vi "Serialize ADAS Data.vi"   [LabVIEW 2020]
uses:
  <vilib>/ADAS Record/CustomDataTypes/ADAS Generic/NI_ADAS_Generic.lvlib
  <vilib>/ADAS Record/CustomDataTypes/Ethernet Type 1/NI_ADAS_Ethernet.lvlib
  <vilib>/ADAS Record/CustomDataTypes/Vision Type 1/NI_ADAS_IMAQ_Array.lvlib
  <vilib>/ADAS Record/CustomDataTypes/CAN/NI_ADAS_CAN.lvlib
  <vilib>/ADAS Record/CustomDataTypes/Audio Data/Audio Data.lvlib
  <vilib>/ADAS Record/CustomDataTypes/Byte Array/Byte Array.lvlib
  <vilib>/ADAS Record/CustomDataTypes/Byte Array EDVR/Byte Array EDVR.lvlib
  <vilib>/ADAS Record/CustomDataTypes/Double/Double.lvlib
  <vilib>/ADAS Record/CustomDataTypes/Ethernet Frame/Ethernet Frame.lvlib
  <vilib>/ADAS Record/CustomDataTypes/Extended (EXT)/Extended (EXT).lvlib
  <vilib>/ADAS Record/CustomDataTypes/LIN Frame Array/LIN Frame Array.lvlib
  <vilib>/ADAS Record/CustomDataTypes/Signed Byte (I8)/Signed Byte (I8).lvlib
  <vilib>/ADAS Record/CustomDataTypes/Signed Long (I32)/Signed Long (I32).lvlib
  <vilib>/ADAS Record/CustomDataTypes/Signed Quad (I64)/Signed Quad (I64).lvlib
  <vilib>/ADAS Record/CustomDataTypes/Signed Word (I16)/Signed Word (I16).lvlib
  <vilib>/ADAS Record/CustomDataTypes/Single/Single.lvlib
  <vilib>/ADAS Record/CustomDataTypes/String/String.lvlib
  <vilib>/ADAS Record/CustomDataTypes/Unsigned Byte (U8)/Unsigned Byte (U8).lvlib
  <vilib>/ADAS Record/CustomDataTypes/Unsigned Long (U32)/Unsigned Long (U32).lvlib
  <vilib>/ADAS Record/CustomDataTypes/Unsigned Quad (U64)/Unsigned Quad (U64).lvlib
  <vilib>/ADAS Record/CustomDataTypes/Unsigned Word (U16)/Unsigned Word (U16).lvlib
  <vilib>/ADAS Record/CustomDataTypes/Integer Waveform (U8)/Integer Waveform (U8).lvlib
  <vilib>/ADAS Record/CustomDataTypes/GPS/GPS.lvlib
  <vilib>/ADAS Record/CustomDataTypes/Waveform(DBL) Array/Waveform(DBL) Array.lvlib
  <vilib>/ADAS Record/CustomDataTypes/Boolean/Boolean.lvlib
  <vilib>/ADAS Record/CustomDataTypes/CameraLLPPacketFIFO/CameraLLPPacketFIFO.lvlib
  <vilib>/ADAS Record/CustomDataTypes/Optitrack/Optitrack.lvlib
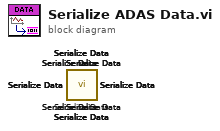
[diagram p0: block diagram]
diagram:
  n1 = call <vilib>:"Serialize Data.vi"() -> ()  [unwired: 10 in, 2 out]
  n2 = call <vilib>:"Serialize Data.vi"() -> ()  [unwired: 10 in, 2 out]
  n3 = call <vilib>:"Serialize Data.vi"() -> ()  [unwired: 10 in, 2 out]
  n4 = call <vilib>:"Serialize Data.vi"() -> ()  [unwired: 10 in, 2 out]
  n5 = call <vilib>:"Serialize Data.vi"() -> ()  [unwired: 10 in, 2 out]
  n6 = call <vilib>:"Serialize Data.vi"() -> ()  [unwired: 10 in, 2 out]
  n7 = call <vilib>:"Serialize Data.vi"() -> ()  [unwired: 10 in, 2 out]
  n8 = call <vilib>:"Serialize Data.vi"() -> ()  [unwired: 10 in, 2 out]
  n9 = call <vilib>:"Serialize Data.vi"() -> ()  [unwired: 10 in, 2 out]
  n10 = call <vilib>:"Serialize Data.vi"() -> ()  [unwired: 10 in, 2 out]
  n11 = call <vilib>:"Serialize Data.vi"() -> ()  [unwired: 10 in, 2 out]
  n12 = call <vilib>:"Serialize Data.vi"() -> ()  [unwired: 10 in, 2 out]
  n13 = call <vilib>:"Serialize Data.vi"() -> ()  [unwired: 10 in, 2 out]
  n14 = call <vilib>:"Serialize Data.vi"() -> ()  [unwired: 10 in, 2 out]
  n15 = call <vilib>:"Serialize Data.vi"() -> ()  [unwired: 10 in, 2 out]
  n16 = call <vilib>:"Serialize Data.vi"() -> ()  [unwired: 10 in, 2 out]
  n17 = call <vilib>:"Serialize Data.vi"() -> ()  [unwired: 10 in, 2 out]
  n18 = call <vilib>:"Serialize Data.vi"() -> ()  [unwired: 10 in, 2 out]
  n19 = call <vilib>:"Serialize Data.vi"() -> ()  [unwired: 10 in, 2 out]
  n20 = call <vilib>:"Serialize Data.vi"() -> ()  [unwired: 10 in, 2 out]
  n21 = call <vilib>:"Serialize Data.vi"() -> ()  [unwired: 10 in, 2 out]
  n22 = call <vilib>:"Serialize Data.vi"() -> ()  [unwired: 10 in, 2 out]
  n23 = call <vilib>:"Serialize Data.vi"() -> ()  [unwired: 10 in, 2 out]
  n24 = call <vilib>:"Serialize Data.vi"() -> ()  [unwired: 10 in, 2 out]
  n25 = call <vilib>:"Serialize Data.vi"() -> ()  [unwired: 10 in, 2 out]
  n26 = call <vilib>:"Serialize Data.vi"() -> ()  [unwired: 10 in, 2 out]
  n27 = call <vilib>:"Serialize Data.vi"() -> ()  [unwired: 10 in, 2 out]
